vi "COD电极校准.vi"() -> ()   [LabVIEW 2016, in "斯坦道多参数.lvlib"]
uses:
  <vilib>/Utility/miscctls.llb/LVPointTypeDef.ctl
  <vilib>/Utility/miscctls.llb/LVPositionTypeDef.ctl
  <vilib>/Analysis/NI_AALBase.lvlib
panel:
  out "COD水样校正值":dbl format="%#.2f"
  out "浊度测量值":dbl format="%#.2f"
  out "浊度信号值":dbl format="%#.2f"
  out "滤波设定":dbl
  in  "刷新按钮":bool
  out "第三点信号值":dbl
  out "第二点信号值":dbl
  out "第一点信号值":dbl
  out "温度":dbl format="%#.2f"
  out "通讯状态":string
  out "第三点校准值":dbl
  out "标液3":dbl
  out "第二点校准值":dbl
  out "第一点校准值":dbl
  in  "校准停止":bool
  in  "校准启动":bool
  in  "校准模式":u16(ring) items=["两点校准", "单点校准", "三点校准"]
  out "最小值":sgl format="%#.2f"
  out "最大值":sgl format="%#.2f"
  out "波形图表":sgl(graph) caption="历史曲线"
  out "mean":dbl caption="均值" format="%#.2f"
  out "standard deviation":dbl caption="标准差" format="%#.2f"
  out "变异系数":dbl format="%#.6f"
  out "COD测量值":dbl format="%#.2f"
  out "提示":string
  out "标液2":dbl
  out "标液1":dbl
  out "COD信号值":dbl format="%#.2f"
  out "COD偏移修正值":dbl format="%#.2f"
  # "COD电极设定"
  # "℃"
  # "请选择校准模式:"
  # "mg/L"
  # "mg/L"
  # "mg/L"
  # "mg/L"
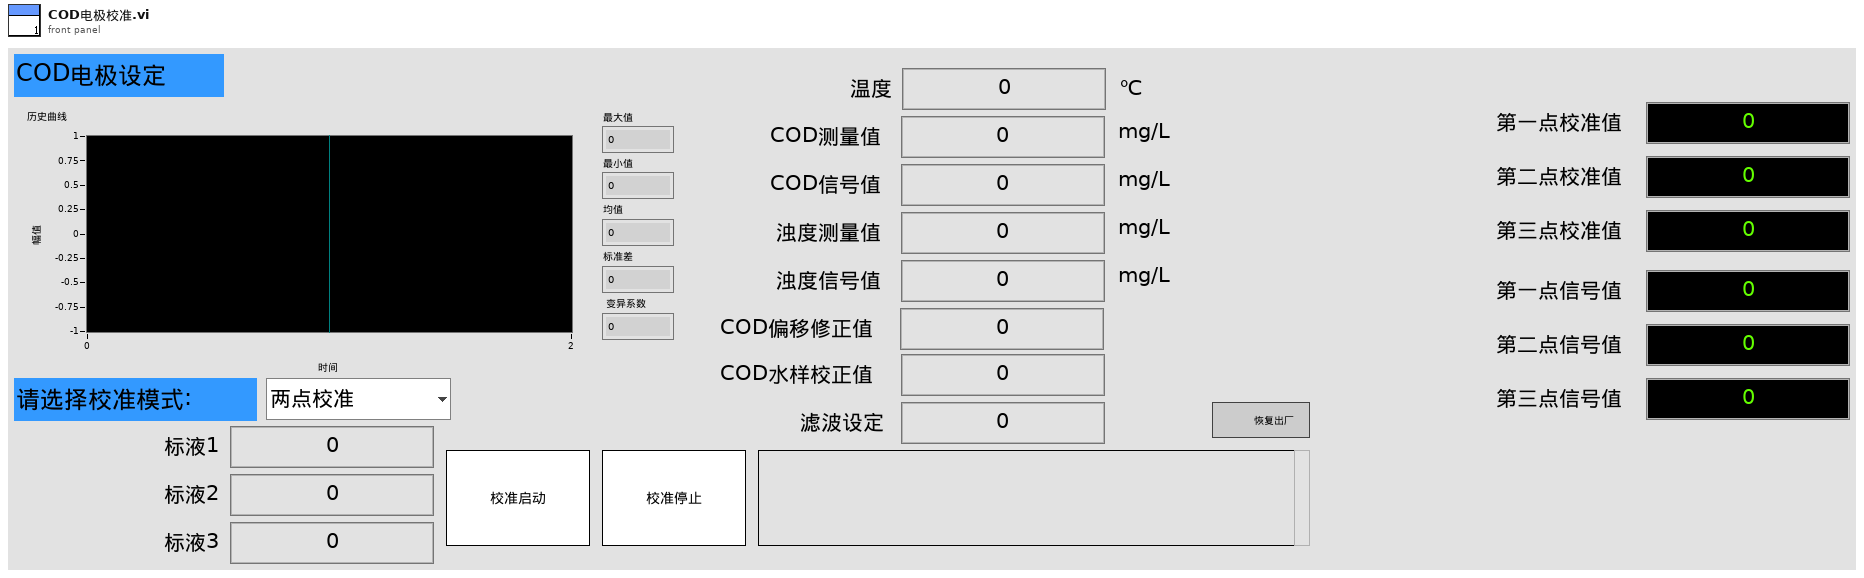
[diagram p1: front panel]
types:
  T1 = enum16{"pH", "DO", "Cond", "Turb", "ORP", "叶绿素a", "藻密度", "COD"}
  T2 = typedef "LVPointTypeDef.ctl" = cluster{"Horizontal":i16, "Vertical":i16}
  T3 = cluster{"电极状态标志":u16, "电极型号标志":u16, "COD测量值":sgl, "浊度测量值":sgl, "COD信号值":sgl, "浊度信号值":sgl, "温度测量值":sgl, "COD偏移修正值":sgl, "浊度偏移修正值":sgl, "COD水样校正值":sgl, "温度偏移修正值":sgl, "COD零点系数":sgl, "COD斜率系数":sgl, "浊度零点系数":sgl, "浊度斜率系数":sgl, "COD测值K值":sgl, "浊度测值K值":sgl, "浊度补偿COD系数值":sgl, "COD温度补偿系数值 ":sgl, "测量周期":u16, "清洗周期":u16, "命令寄存器":u16, "数字滤波设定":u16, "温度模式":enum16{"AUTO", "OFF"}, "生产批次":u16, "电极序号":u16, "串口地址":u16, "串口波特率":enum16{"9600", "19200", "115200"}, "串口校验位":enum16{"NONE", "ODD", "EVEN"}, "串口停止位":enum16{"1bit", "2bit"}, "第一点校正指令":u16, "第一点标准值":sgl, "第二点校正指令":u16, "第二点标准值":sgl, "第三点校正指令":u16, "第三点标准值":sgl, "COD吸光度":sgl, "浊度吸光度":sgl, "温度信号值":sgl}
  T4 = typedef "LVPositionTypeDef.ctl" = cluster{"Left":i32, "Top":i32}
  T5 = enum8{"Enabled", "Disabled", "Disabled and Grayed Out"}
  T6 = cluster{"测量量程":dbl, "测量精度":dbl, "测量间隔":dbl, "消解温度":dbl, "消解时长":dbl, "空白校准时间":timestamp, "曲线截距":dbl, "曲线斜率":dbl, "测量检出限":dbl, "测量信号值":dbl, "线性相关系数":dbl, "二次多项式系数":dbl, "标样校准时间":timestamp, "稀释倍数":dbl, "三项式系数":dbl, "空白标定系数":dbl, "量程系数":dbl, "F0/ORPA":dbl, "F1/ORPB":dbl, "F2/ORPK":dbl, "F3":dbl, "F4":dbl, "F5":dbl, "F6":dbl, "F7":dbl, "X0/滴定数":dbl, "量程":dbl}
  T7 = cluster{"ph":bool, "DO":bool, "Cond":bool, "Turb":bool, "叶绿素a":bool, "藻密度":bool, "ORP":bool, "COD":bool}
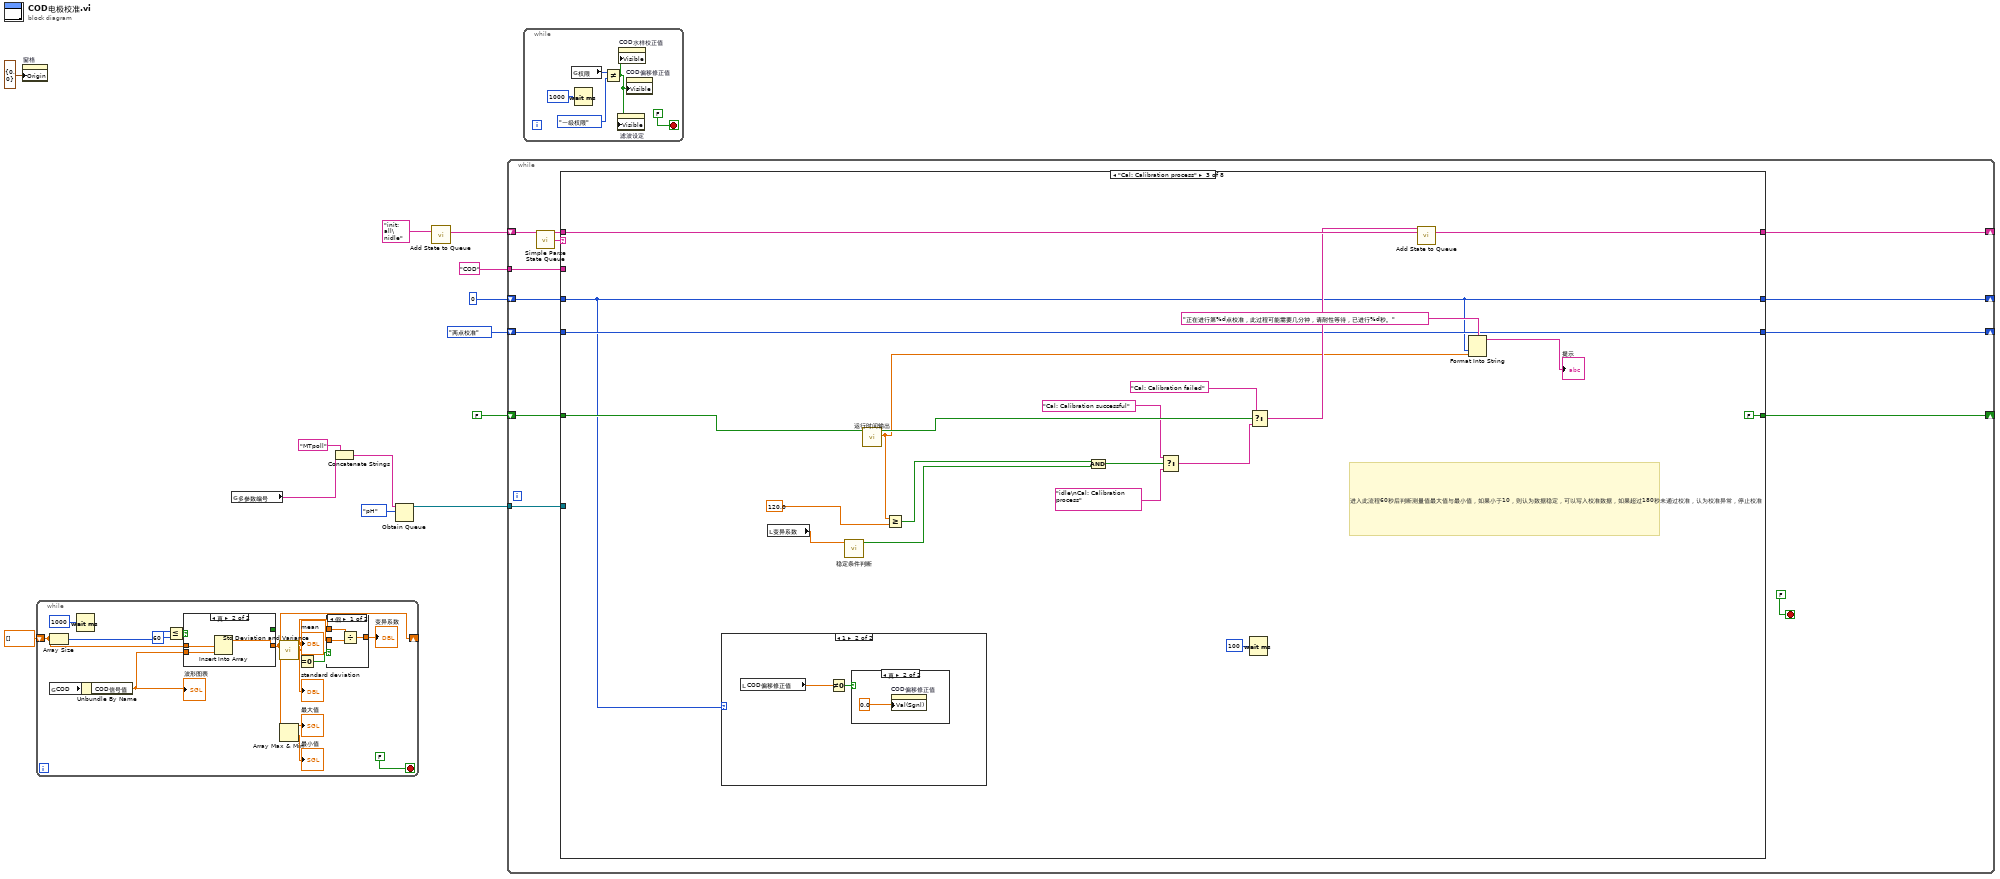
[diagram p0: block diagram]
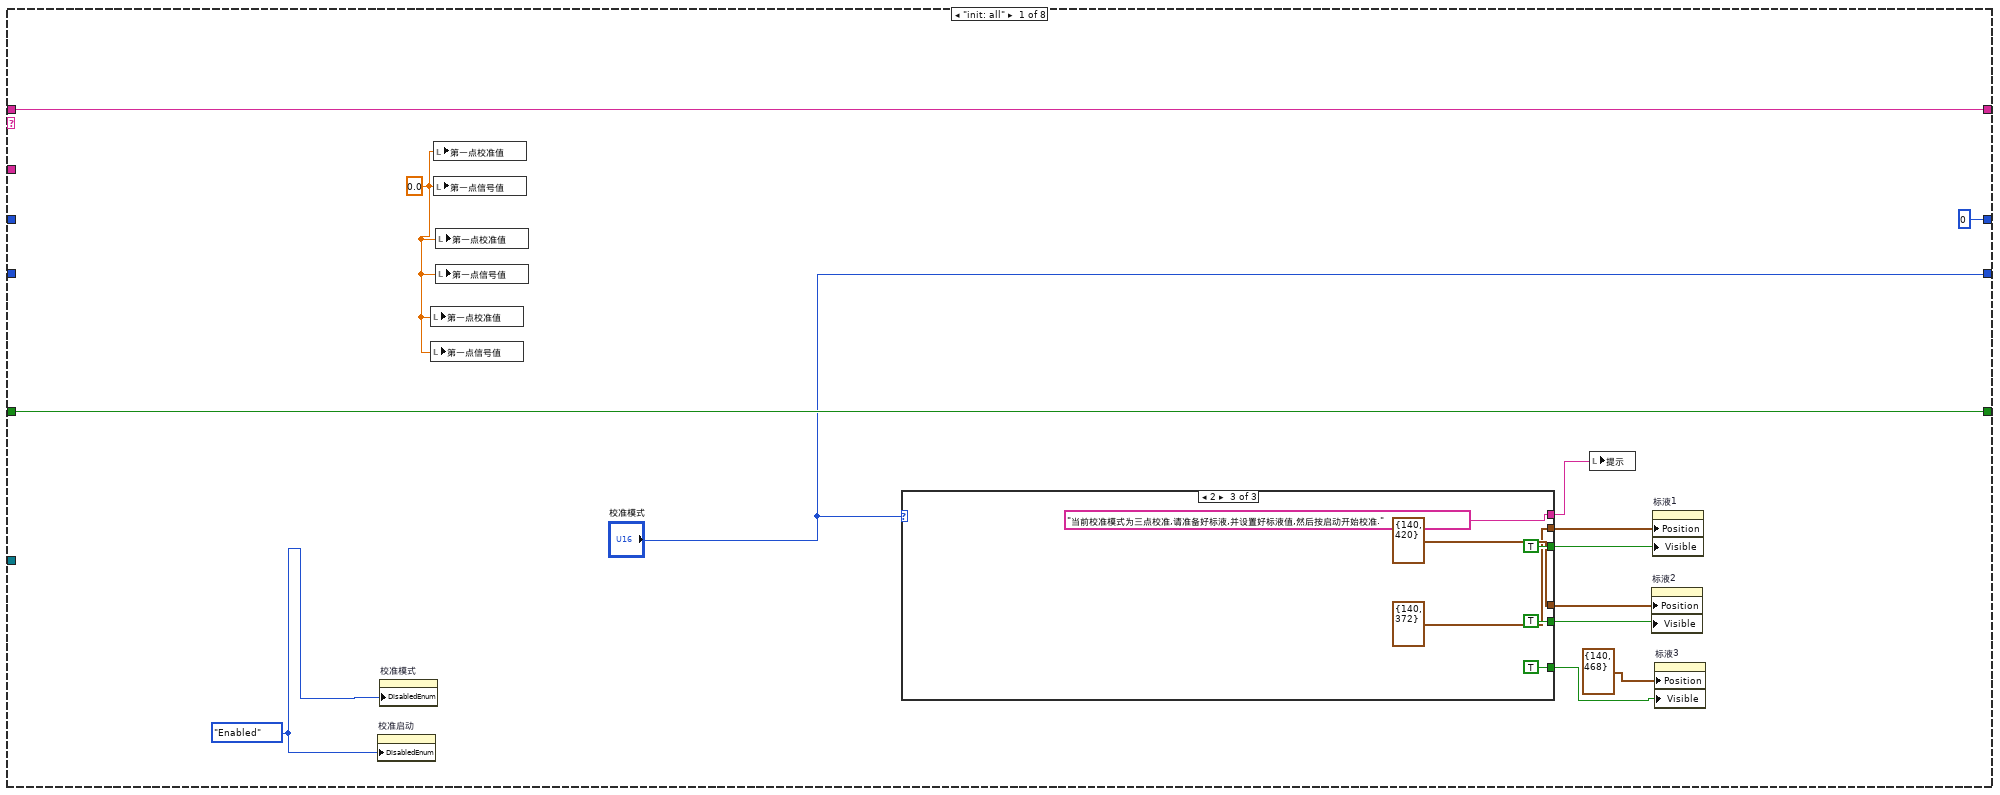
[diagram p2: hidden frame]
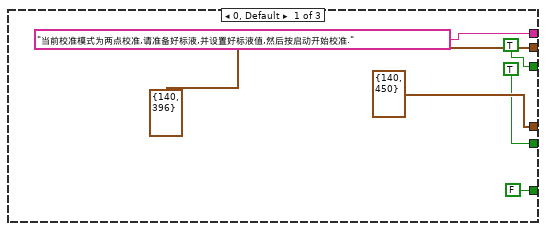
[diagram p3: hidden frame]
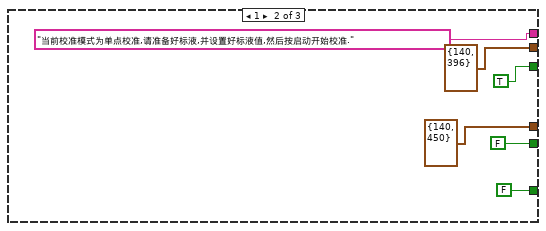
[diagram p4: hidden frame]
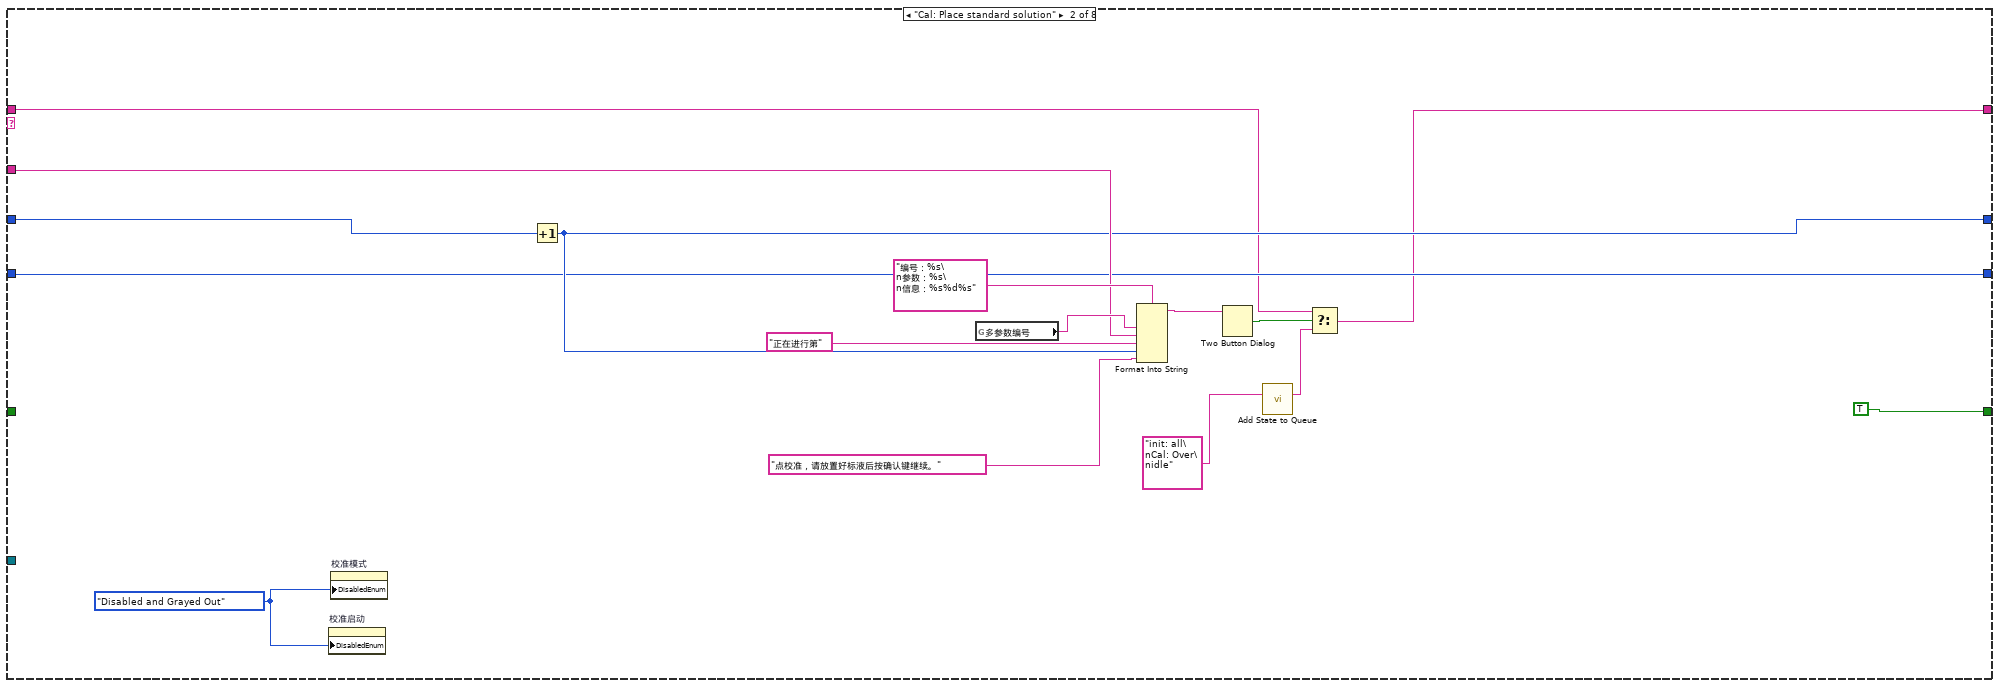
[diagram p5: hidden frame]
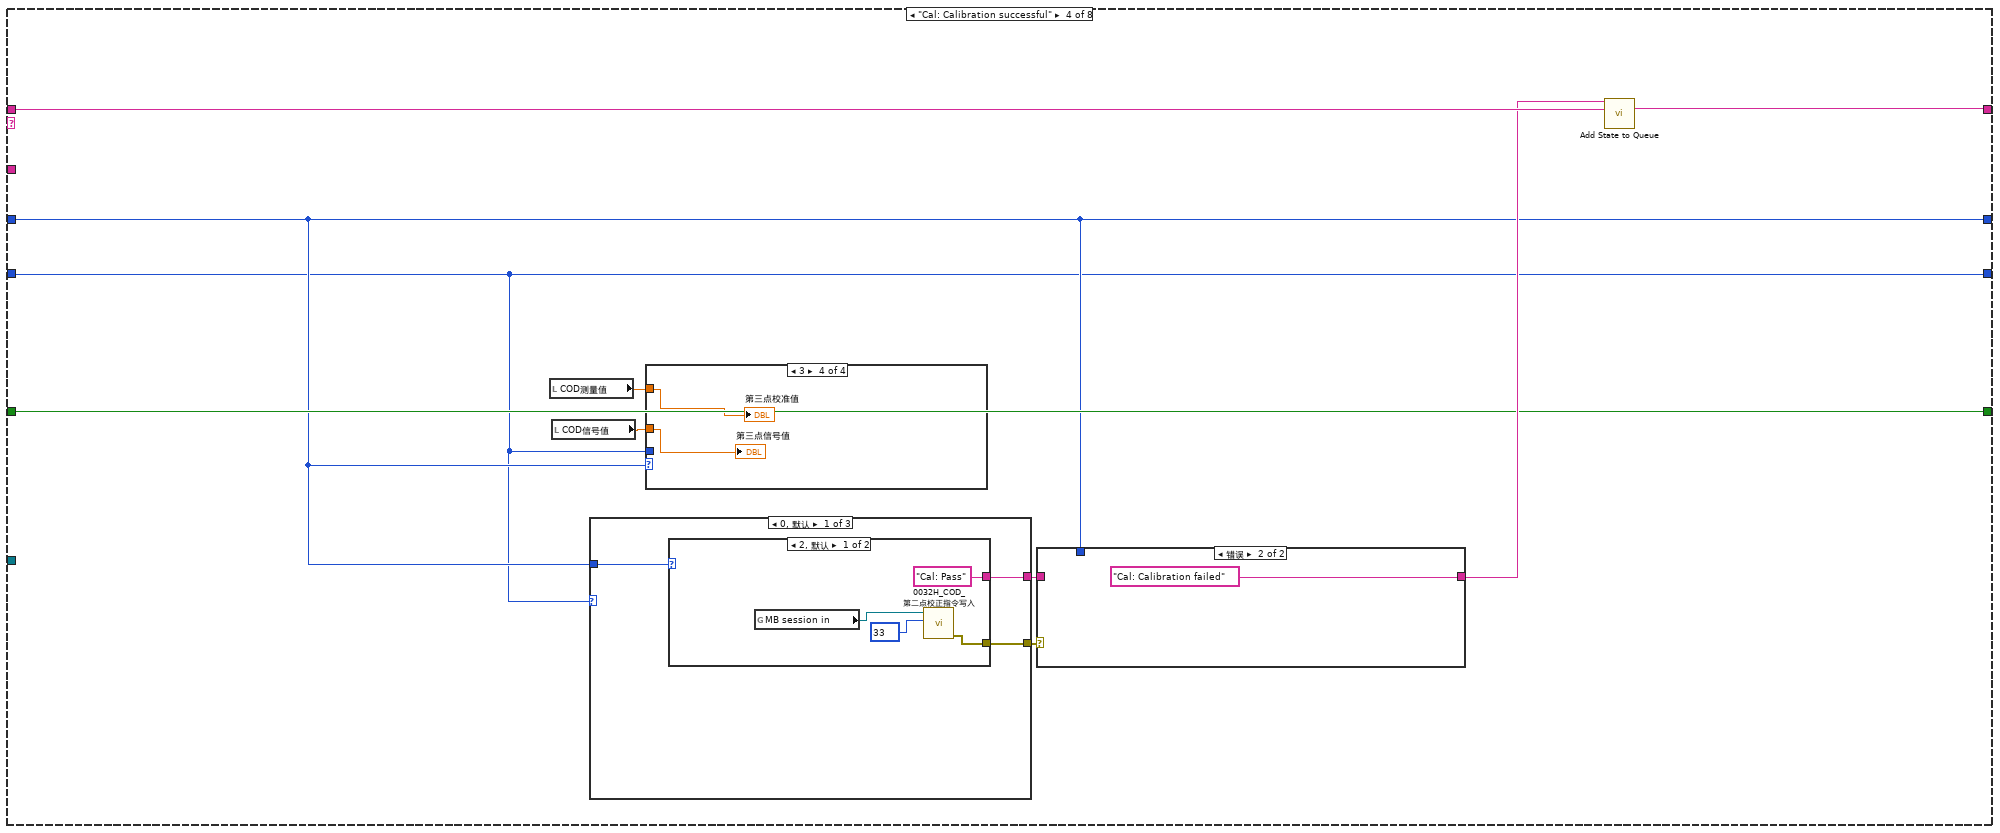
[diagram p8: hidden frame]
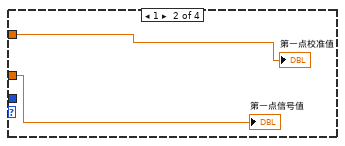
[diagram p10: hidden frame]
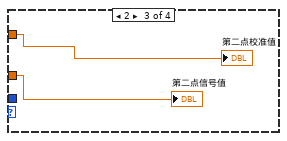
[diagram p11: hidden frame]
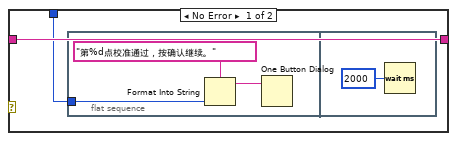
[diagram p12: hidden frame]
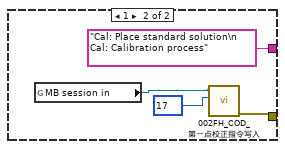
[diagram p13: hidden frame]
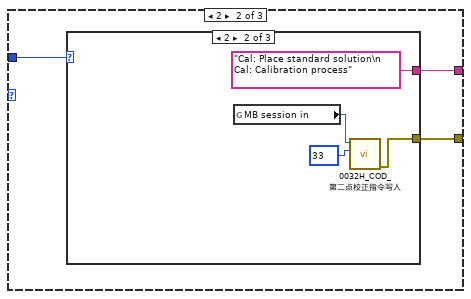
[diagram p14: hidden frame]
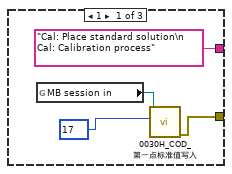
[diagram p15: hidden frame]
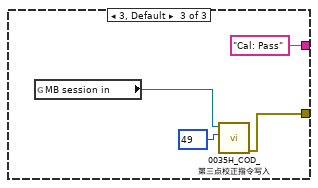
[diagram p16: hidden frame]
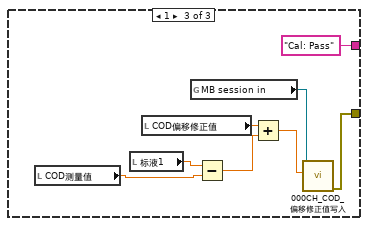
[diagram p17: hidden frame]
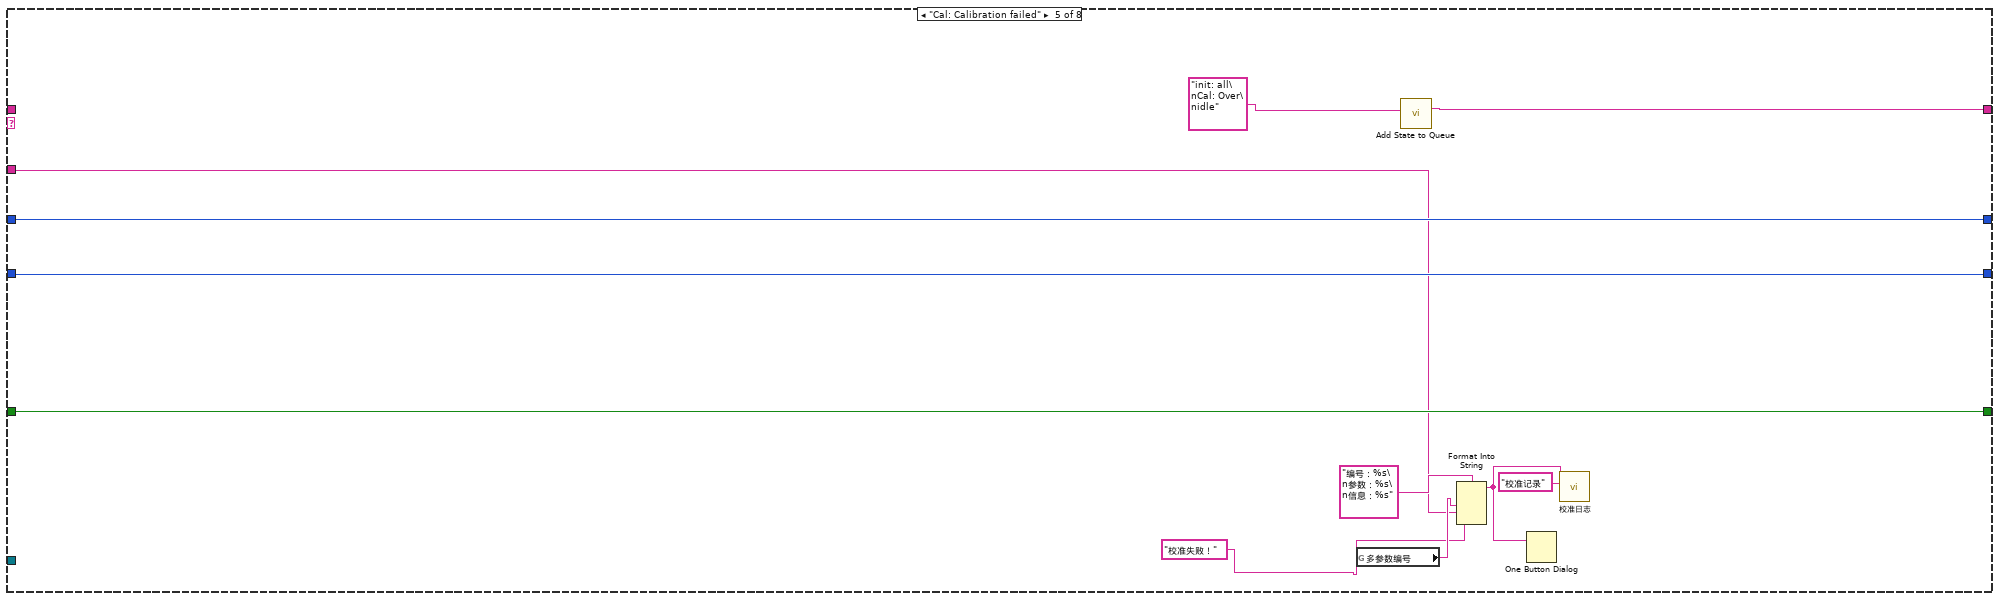
[diagram p18: hidden frame]
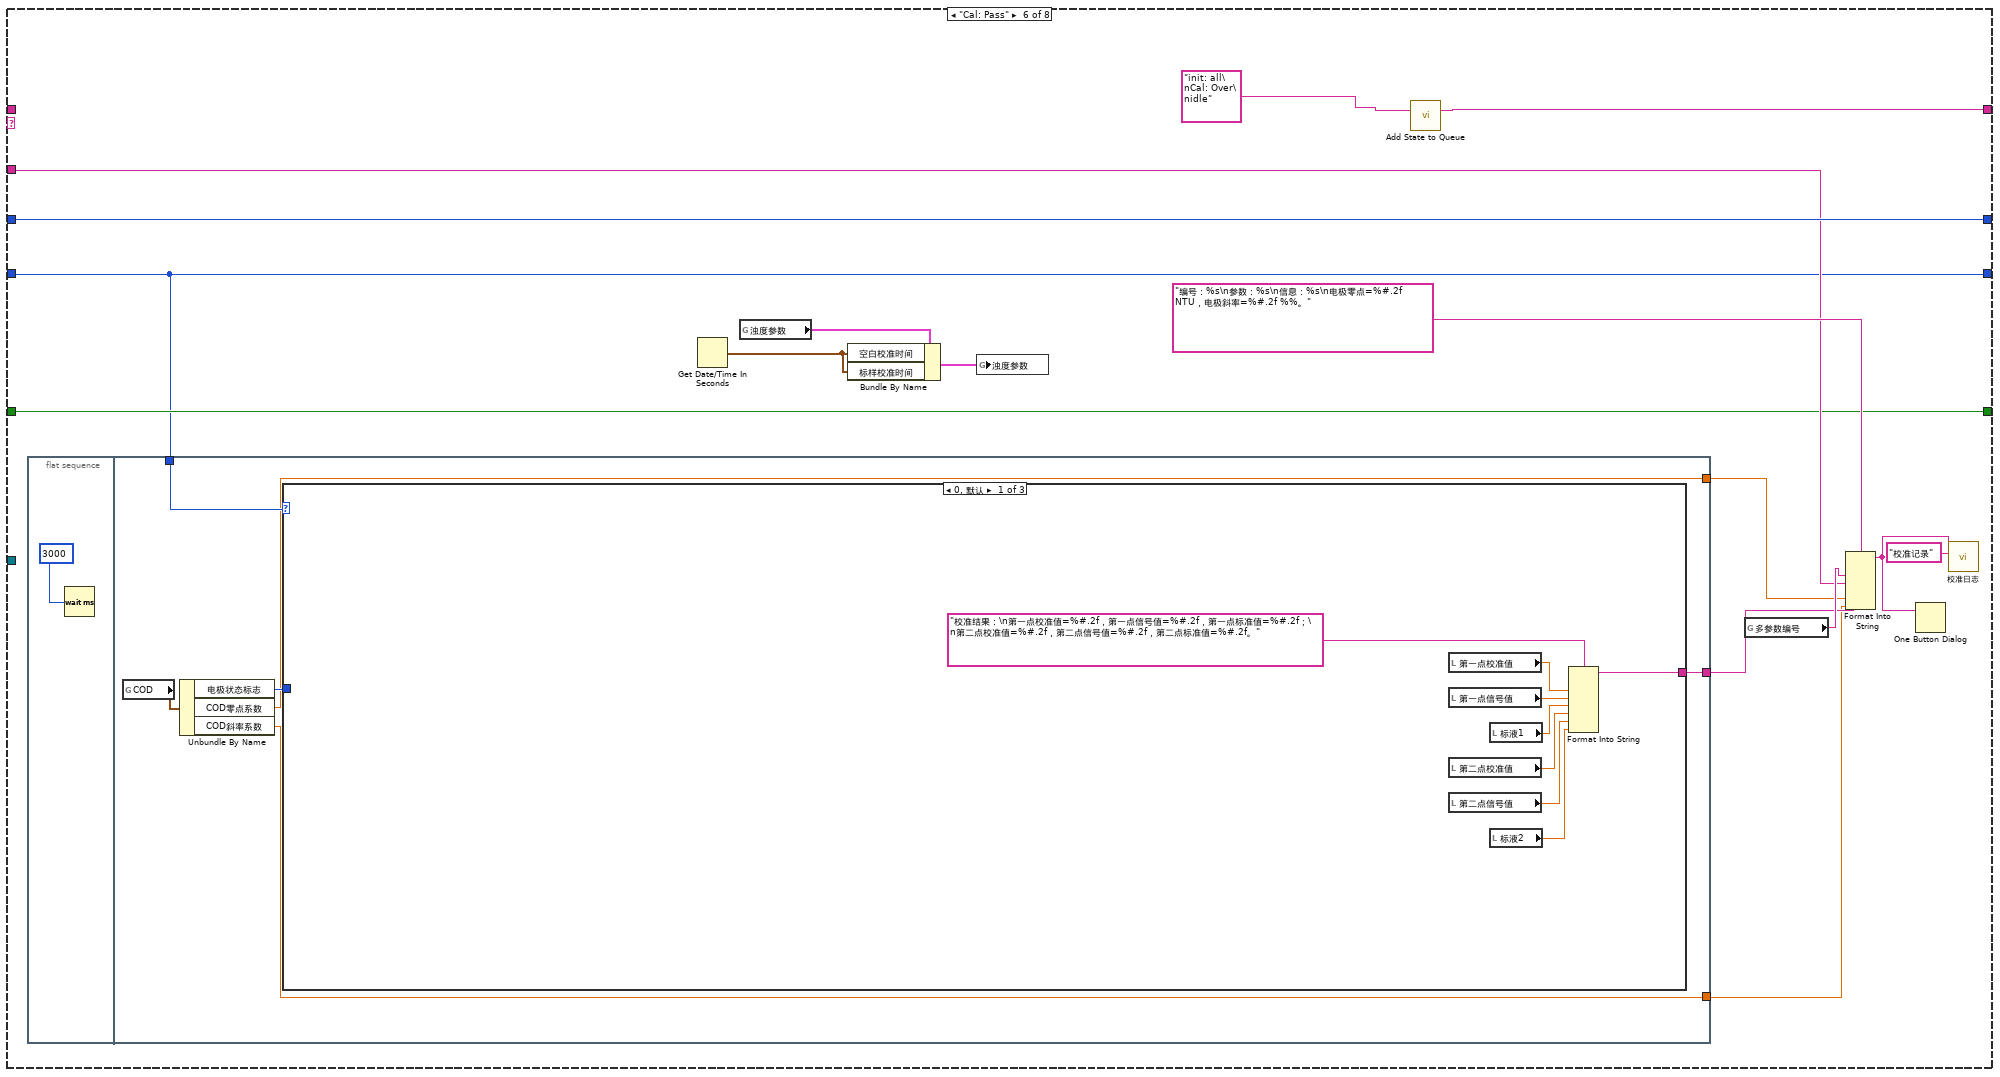
[diagram p19: hidden frame]
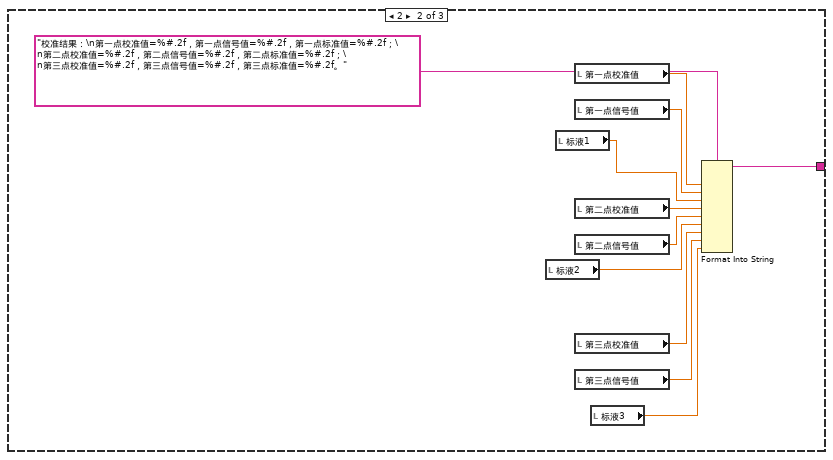
[diagram p20: hidden frame]
diagram:
  n1 = property on="窗格" class="Pane"("Origin"=T2 {"Horizontal"=0, "Vertical"=0} ("原点")) -> ()  [unwired: 2 in, 2 out]
  n2 = while {
    shift-right: [w17] -> _
    shift-left: sgl[] [] -> [w24]
    stop <- FALSE stop-if-true
    n3 = Array Size(array=w24) -> (size(s)=w26:i32)
    n4 = global read "国弘过程全局变量.vi" "COD"() -> (w18:T3)
    n5 = Wait (ms)(milliseconds to wait=u32 1000 ("等待时间（毫秒）")) -> ()  [unwired: 1 out]
    n6 = Unbundle By Name(w18) -> ("COD信号值"=w14:sgl)
    "波形图表" <- w14
    n7 = Less Or Equal?(x=w26, y=60) -> (x <= y?=w25:bool)
    n8 = case shown="真" w25 {
      tunnel: w24 -> [w37 w40]
      tunnel: w14 -> [w35 w39]
      tunnel: [w33 w38] -> w17
      tunnel: [TRUE _] -> _
      frame False {
        n9 = Replace Array Subset(array=w37, new element=w35) -> (w36:sgl[])  [unwired: 1 in]
        n10 = Rotate 1D Array(1:w36, 2:-1 ("n")) -> (0:w33:sgl[])
      }
      frame True {
        n11 = Insert Into Array(array=w40, new element=w39) -> (w38:sgl[])  [unwired: 1 in]
      }
    }
    n12 = call <vilib>:"Std Deviation and Variance.vi"("X"=w17) -> ("mean"=w22:dbl, "standard deviation"=w21:dbl)  [unwired: 1 in, 1 out]
    "mean" <- w22
    "standard deviation" <- w21
    n13 = Array Max & Min(array=w17) -> (max value=→"最大值":sgl, min value=→"最小值":sgl)  [unwired: 2 out]
    n14 = Equal To 0?(x=w22) -> (x = 0?=w23:bool)
    n15 = case shown="假" w23 {
      tunnel: w21 -> [w31 _]
      tunnel: [w30 _] -> w20
      tunnel: w22 -> [w29 _]
      frame False {
        n16 = Divide(x=w31, y=w29) -> (x/y=w30:dbl)
      }
      frame True {
      }
    }
    "变异系数" <- w20
  }
  n17 = global read "多参数全局变量.vi" "多参数编号"() -> (w2:string)
  n18 = Concatenate Strings("MTpoll" ("名称（未命名）"), w2) -> (w4:string)
  n19 = Obtain Queue(name (unnamed)=w4, element data type=T1."pH" ("枚举")) -> (queue out=w1:refnum<queue>)  [unwired: 3 in, 2 out]
  n20 = call "Add State to Queue.vi"("State(s) In (\"\")"="init: all\nidle" ("State(s) In (\"\")")) -> ("States Out"=w10:string)  [unwired: 14 in]
  n21 = while {
    shift-right: [w49] -> _
    shift-left: w10 -> [w53]
    shift-right: [w46] -> _
    shift-left: 0 -> [w48]
    tunnel: "COD" ("State(s) In (\"\")") -> [w47]
    shift-right: [w44] -> _
    shift-left: enum16{"两点校准", "单点校准", "三点校准"}."两点校准" ("校准模式") -> [w45]
    shift-right: [w42] -> _
    shift-left: FALSE -> [w43]
    tunnel: w1 -> [w41]
    stop <- FALSE stop-if-true
    n22 = call "Simple Parse State Queue.vi"("State Queue"=w53) -> ("Remain States"=w50:string, "Next State"=w51:string)  [unwired: 13 in]
    n23 = case shown="\"Cal: Calibration process\"" w51 {
      tunnel: w50 -> [w66 w88 w120 w132 _ _ w243 w254]
      tunnel: [w66 w87 w119 w131 w189 w199 w243 w253] -> w49
      tunnel: w48 -> [_ w96 w105 w126 w192 w208 w242 w251]
      tunnel: w47 -> [_ w97 _ _ w183 w204 _ _]
      tunnel: [0 w94 w105 w126 w192 w208 w242 w252] -> w46
      tunnel: w45 -> [_ w93 w106 w125 w191 w200 w241 w250]
      tunnel: ["校准模式" w93 w106 w125 w191 w200 w241 w250] -> w44
      tunnel: w43 -> [w63 _ w108 w127 w190 w203 w240 w248]
      tunnel: [w63 TRUE FALSE w127 w190 w203 w240 w248] -> w42
      tunnel: w41 -> [_ _ _ _ _ _ _ w247]
      frame "init: all" {
        w61 = T5."Enabled" ("禁用")
        w62 = 0.0 ("第一点校准值")
        n24 = property on="校准启动" class="Bool"("DisabledEnum"=w61) -> ()  [unwired: 2 in, 2 out]
        n25 = property on="校准模式" class="Ring (严格)"("DisabledEnum"=w61) -> ()  [unwired: 2 in, 2 out]
        n26 = local write "第一点校准值"(w62) -> ()
        n27 = local write "第一点信号值"(w62) -> ()
        n28 = local write "第一点校准值"(w62) -> ()
        n29 = local write "第一点信号值"(w62) -> ()
        n30 = local write "第一点校准值"(w62) -> ()
        n31 = local write "第一点信号值"(w62) -> ()
        n32 = case shown="2" "校准模式" {
          tunnel: ["当前校准模式为两点校准,请准备好标液,并设置好标液值,然后按启动开始校准." ("提示") "当前校准模式为单点校准,请准备好标液,并设置好标液值,然后按启动开始校准." ("提示") "当前校准模式为三点校准,请准备好标液,并设置好标液值,然后按启动开始校准." ("提示")] -> w65
          tunnel: [T4 {"Left"=140, "Top"=396} ("位置") T4 {"Left"=140, "Top"=396} ("位置") T4 {"Left"=140, "Top"=372} ("位置")] -> w59
          tunnel: [TRUE ("可见") TRUE ("可见") TRUE ("可见")] -> w58
          tunnel: [FALSE ("可见") FALSE ("可见") TRUE ("可见")] -> w56
          tunnel: [TRUE ("可见") FALSE ("可见") TRUE ("可见")] -> w55
          tunnel: [T4 {"Left"=140, "Top"=450} ("位置 2") T4 {"Left"=140, "Top"=450} ("位置 2") T4 {"Left"=140, "Top"=420} ("位置 2")] -> w54
          frame 0, Default {
          }
          frame 1 {
          }
          frame 2 {
          }
        }
        n33 = local write "提示"(w65) -> ()
        n34 = property on="标液2" class="DigNum (严格)"("Position"=w54, "Visible"=w55) -> ()  [unwired: 2 in, 2 out]
        n35 = property on="标液1" class="DigNum (严格)"("Position"=w59, "Visible"=w58) -> ()  [unwired: 2 in, 2 out]
        n36 = property on="标液3" class="DigNum (严格)"("Position"=T4 {"Left"=140, "Top"=468} ("位置 3"), "Visible"=w56) -> ()  [unwired: 2 in, 2 out]
      }
      frame "Cal: Place standard solution" {
        w86 = T5."Disabled and Grayed Out" ("禁用")
        n37 = property on="校准启动" class="Bool"("DisabledEnum"=w86) -> ()  [unwired: 2 in, 2 out]
        n38 = property on="校准模式" class="Ring (严格)"("DisabledEnum"=w86) -> ()  [unwired: 2 in, 2 out]
        n39 = Increment(x=w96) -> (x+1=w94:i32)
        n40 = global read "多参数全局变量.vi" "多参数编号"() -> (w99:string)
        n41 = Format Into String(format string="编号：%s\n参数：%s\n信息：%s%d%s" ("格式字符串"), w99, w97, "正在进行第" ("消息"), w94, "点校准，请放置好标液后按确认键继续。" ("消息")) -> (resulting string=w91:string)  [unwired: 2 in, 1 out]
        n42 = Two Button Dialog(message=w91) -> (T button?=w90:bool)  [unwired: 2 in]
        n43 = call "Add State to Queue.vi"("State(s) In (\"\")"="init: all\nCal: Over\nidle" ("State(s) In (\"\")")) -> ("States Out"=w89:string)  [unwired: 14 in]
        n44 = Select(t=w88, s=w90, f=w89) -> (s? t:f=w87:string)
      }
      frame "Cal: Calibration process" {
        # "进入此流程60秒后判断测量值最大值与最小值，如果小于10，则认为数据稳定，可以写入校准数据，如果超过180秒未通过校准，认为校准异常，停止校准"
        n45 = case shown="1" w105 {
          frame 0, Default {
          }
          frame 1 {
            n46 = local read "COD偏移修正值"() -> (w122:dbl)
            n47 = Not Equal To 0?(x=w122) -> (x != 0?=w123:bool)
            n48 = case shown="真" w123 {
              frame False {
              }
              frame True {
                n49 = property on="COD偏移修正值" class="DigNum (严格)"("Val(Sgnl)"=0.0 ("值(信号)")) -> ()  [unwired: 2 in, 2 out]
              }
            }
          }
        }
        n50 = local read "变异系数"() -> (w102:dbl)
        n51 = call "稳定条件判断.vi"("变异系数"=w102) -> ("布尔"=w101:bool)  [unwired: 10 in]
        n52 = call "运行时间输出.vi"("初始化"=w108) -> ("Elapsed Time (s)"=w104:dbl, "Time has Elapsed"=w121:bool)  [unwired: 9 in]
        n53 = Greater Or Equal?(x=w104, y=120.0) -> (x >= y?=w116:bool)
        n54 = And(x=w116, y=w101) -> (x .and. y?=w113:bool)
        n55 = Select(t="Cal: Calibration successful" ("State(s) In (\"\")"), s=w113, f="idle\nCal: Calibration process" ("State(s) In (\"\")")) -> (s? t:f=w112:string)
        n56 = Wait (ms)(milliseconds to wait=u32 100 ("等待时间（毫秒）")) -> ()  [unwired: 1 out]
        n57 = Select(t="Cal: Calibration failed" ("State(s) In (\"\")"), s=w121, f=w112) -> (s? t:f=w111:string)
        n58 = call "Add State to Queue.vi"("State(s) In Front (\"\")"=w111, "State(s) In (\"\")"=w120) -> ("States Out"=w119:string)  [unwired: 13 in]
        n59 = Format Into String(format string="正在进行第%d点校准，此过程可能需要几分钟，请耐性等待，已进行%d秒。" ("格式字符串"), w105, w104) -> (resulting string=→"提示":string)  [unwired: 2 in, 1 out]
      }
      frame "Cal: Calibration successful" {
        n60 = local read "COD测量值"() -> (w128:dbl)
        n61 = local read "COD信号值"() -> (w129:dbl)
        n62 = case shown="0, 默认" w125 {
          tunnel: [w150 w161 w174] -> w134
          tunnel: [w149 w159 "Cal: Pass" ("State(s) In (\"\")")] -> w133
          tunnel: w126 -> [w148 w160 _]
          frame 0, Default {
            n63 = case shown="2, 默认" w148 {
              tunnel: [w153 w157] -> w150
              tunnel: ["Cal: Pass" ("State(s) In (\"\")") "Cal: Place standard solution\n Cal: Calibration process" ("State(s) In (\"\")")] -> w149
              frame 2, Default {
                n64 = global read "多参数全局变量.vi" "MB session in"() -> (w152:refnum<class "MB_Master.lvclass">)
                n65 = call "0032H_COD_第二点校正指令写入.vi"("数值"=u16 33, "MB session in"=w152) -> ("error out"=w153:errorcluster)  [unwired: 8 in, 1 out]
              }
              frame 1 {
                n66 = global read "多参数全局变量.vi" "MB session in"() -> (w156:refnum<class "MB_Master.lvclass">)
                n67 = call "002FH_COD_第一点校正指令写入.vi"("数值"=u16 17, "MB session in"=w156) -> ("error out"=w157:errorcluster)  [unwired: 8 in, 1 out]
              }
            }
          }
          frame 2 {
            n68 = case shown="2" w160 {
              tunnel: [w164 w167 w171] -> w161
              tunnel: ["Cal: Place standard solution\n Cal: Calibration process" ("State(s) In (\"\")") "Cal: Place standard solution\n Cal: Calibration process" ("State(s) In (\"\")") "Cal: Pass" ("State(s) In (\"\")")] -> w159
              frame 1 {
                n69 = global read "多参数全局变量.vi" "MB session in"() -> (w163:refnum<class "MB_Master.lvclass">)
                n70 = call "0030H_COD_第一点标准值写入.vi"("数值"=u16 17, "MB session in"=w163) -> ("error out"=w164:errorcluster)  [unwired: 8 in, 1 out]
              }
              frame 2 {
                n71 = global read "多参数全局变量.vi" "MB session in"() -> (w166:refnum<class "MB_Master.lvclass">)
                n72 = call "0032H_COD_第二点校正指令写入.vi"("数值"=u16 33, "MB session in"=w166) -> ("error out"=w167:errorcluster)  [unwired: 8 in, 1 out]
              }
              frame 3, Default {
                n73 = global read "多参数全局变量.vi" "MB session in"() -> (w170:refnum<class "MB_Master.lvclass">)
                n74 = call "0035H_COD_第三点校正指令写入.vi"("数值"=u16 49, "MB session in"=w170) -> ("error out"=w171:errorcluster)  [unwired: 8 in, 1 out]
              }
            }
          }
          frame 1 {
            n75 = local read "COD测量值"() -> (w177:dbl)
            n76 = local read "标液1"() -> (w181:dbl)
            n77 = local read "COD偏移修正值"() -> (w179:dbl)
            n78 = global read "多参数全局变量.vi" "MB session in"() -> (w176:refnum<class "MB_Master.lvclass">)
            n79 = Subtract(x=w181, y=w177) -> (x-y=w180:dbl)
            n80 = Add(x=w179, y=w180) -> (x+y=w175:dbl)
            n81 = call "000CH_COD_偏移修正值写入.vi"("数值"=w175, "MB session in"=w176) -> ("error out"=w174:errorcluster)  [unwired: 8 in, 1 out]
          }
        }
        n82 = case shown="3" w126 {
          tunnel: w129 -> [_ w136 w138 w140]
          tunnel: w128 -> [_ w135 w137 w139]
          tunnel: w125 -> [_ _ _ _]
          frame 0, Default {
          }
          frame 1 {
            "第一点信号值" <- w136
            "第一点校准值" <- w135
          }
          frame 2 {
            "第二点信号值" <- w138
            "第二点校准值" <- w137
          }
          frame 3 {
            "第三点信号值" <- w140
            "第三点校准值" <- w139
          }
        }
        n83 = case shown="错误" w134 {
          tunnel: w133 -> [w142 _]
          tunnel: [w142 "Cal: Calibration failed" ("State(s) In (\"\")")] -> w130
          tunnel: w126 -> [w141 _]
          frame No Error {
            n84 = flat-sequence {
              tunnel: w141 -> [w143]
              frame #0 {
                n85 = Format Into String(format string="第%d点校准通过，按确认继续。" ("格式字符串"), w143) -> (resulting string=w145:string)  [unwired: 2 in, 1 out]
                n86 = One Button Dialog(message=w145) -> ()  [unwired: 1 in, 1 out]
              }
              frame #1 {
                n87 = Wait (ms)(milliseconds to wait=u32 2000 ("等待时间（毫秒）")) -> ()  [unwired: 1 out]
              }
            }
          }
          frame Error {
          }
        }
        n88 = call "Add State to Queue.vi"("State(s) In Front (\"\")"=w130, "State(s) In (\"\")"=w132) -> ("States Out"=w131:string)  [unwired: 13 in]
      }
      frame "Cal: Calibration failed" {
        n89 = global read "多参数全局变量.vi" "多参数编号"() -> (w186:string)
        n90 = call "Add State to Queue.vi"("State(s) In (\"\")"="init: all\nCal: Over\nidle" ("State(s) In (\"\")")) -> ("States Out"=w189:string)  [unwired: 14 in]
        n91 = Format Into String(format string="编号：%s\n参数：%s\n信息：%s" ("格式字符串"), w186, w183, "校准失败！" ("消息")) -> (resulting string=w185:string)  [unwired: 2 in, 1 out]
        n92 = One Button Dialog(message=w185) -> ()  [unwired: 1 in, 1 out]
        n93 = call "校准日志.vi"("table"="校准记录", "日志信息"=w185) -> ()  [unwired: 9 in, 1 out]
      }
      frame "Cal: Pass" {
        n94 = flat-sequence {
          tunnel: [w213] -> w201
          tunnel: w200 -> [w212]
          tunnel: [w211] -> w198
          tunnel: [w210] -> w197
          frame #0 {
            n95 = Wait (ms)(milliseconds to wait=u32 3000 ("等待时间（毫秒）")) -> ()  [unwired: 1 out]
          }
          frame #1 {
            n96 = global read "国弘过程全局变量.vi" "COD"() -> (w214:T3)
            n97 = Unbundle By Name(w214) -> ("电极状态标志"=w215:u16, "COD零点系数"=w211:sgl, "COD斜率系数"=w210:sgl)
            n98 = case shown="0, 默认" w212 {
              tunnel: [w223 w234 w239] -> w213
              tunnel: w215 -> [_ _ _]
              frame 0, Default {
                n99 = local read "第一点校准值"() -> (w221:dbl)
                n100 = local read "第一点信号值"() -> (w222:dbl)
                n101 = local read "第二点校准值"() -> (w218:dbl)
                n102 = local read "第二点信号值"() -> (w217:dbl)
                n103 = local read "标液1"() -> (w219:dbl)
                n104 = local read "标液2"() -> (w216:dbl)
                n105 = Format Into String(format string="校准结果：\n第一点校准值=%#.2f，第一点信号值=%#.2f，第一点标准值=%#.2f；\n第二点校准值=%#.2f，第二点信号值=%#.2f，第二点标准值=%#.2f。" ("提示"), w221, w222, w219, w218, w217, w216) -> (resulting string=w223:string)  [unwired: 2 in, 1 out]
              }
              frame 2 {
                n106 = local read "标液2"() -> (w225:dbl)
                n107 = local read "标液1"() -> (w226:dbl)
                n108 = local read "第一点校准值"() -> (w233:dbl)
                n109 = local read "第一点信号值"() -> (w231:dbl)
                n110 = local read "第二点校准值"() -> (w230:dbl)
                n111 = local read "第二点信号值"() -> (w229:dbl)
                n112 = local read "第三点校准值"() -> (w228:dbl)
                n113 = local read "第三点信号值"() -> (w227:dbl)
                n114 = local read "标液3"() -> (w224:dbl)
                n115 = Format Into String(format string="校准结果：\n第一点校准值=%#.2f，第一点信号值=%#.2f，第一点标准值=%#.2f；\n第二点校准值=%#.2f，第二点信号值=%#.2f，第二点标准值=%#.2f；\n第三点校准值=%#.2f，第三点信号值=%#.2f，第三点标准值=%#.2f。" ("提示"), w233, w231, w226, w230, w229, w225, w228, w227, w224) -> (resulting string=w234:string)  [unwired: 2 in, 1 out]
              }
              frame 1 {
                n116 = local read "第一点校准值"() -> (w238:dbl)
                n117 = local read "第一点信号值"() -> (w236:dbl)
                n118 = local read "标液1"() -> (w235:dbl)
                n119 = Format Into String(format string="校准结果：\n校准值=%#.2f，信号值=%#.2f，标准值=%#.2f。" ("提示"), w238, w236, w235) -> (resulting string=w239:string)  [unwired: 2 in, 1 out]
              }
            }
          }
        }
        n120 = Get Date/Time In Seconds() -> (seconds since 1Jan1904=w193:timestamp)
        n121 = global read "断电保存变量.vi" "浊度参数"() -> (w195:T6)
        n122 = Bundle By Name(cluster=w195, "空白校准时间"=w193, "标样校准时间"=w193) -> (w194:T6)
        n123 = global write "断电保存变量.vi" "浊度参数"(w194) -> ()
        n124 = call "Add State to Queue.vi"("State(s) In (\"\")"="init: all\nCal: Over\nidle" ("State(s) In (\"\")")) -> ("States Out"=w199:string)  [unwired: 14 in]
        n125 = global read "多参数全局变量.vi" "多参数编号"() -> (w205:string)
        n126 = Format Into String(format string="编号：%s\n参数：%s\n信息：%s\n电极零点=%#.2f NTU，电极斜率=%#.2f %%。" ("格式字符串"), w205, w204, w201, w198, w197) -> (resulting string=w202:string)  [unwired: 2 in, 1 out]
        n127 = One Button Dialog(message=w202) -> ()  [unwired: 1 in, 1 out]
        n128 = call "校准日志.vi"("table"="校准记录", "日志信息"=w202) -> ()  [unwired: 9 in, 1 out]
      }
      frame "Cal: Over" {
        n129 = global read "多参数全局变量.vi" "校准运行状态"() -> (w245:T7)
        n130 = Bundle By Name(cluster=w245, "COD"=FALSE ("Turb")) -> (w246:T7)
        n131 = global write "多参数全局变量.vi" "校准运行状态"(w246) -> ()
      }
      frame "idle", Default {
        n132 = event shown="[0] 超时" {
          selector: _ -> [_ _ _ _ _ _ _ _ _ _ _ _]
          dyn-events: _ -> [_ _ _ _ _ _ _ _ _ _ _ _]
          timeout: 10 -> [_ _ _ _ _ _ _ _ _ _ _ _]
          tunnel: [_ _ _ w287 w296 w305 w314 w323 w332 _ _ _] -> _
          tunnel: w254 -> [w273 w277 w282 w293 w302 w306 w315 w324 w336 w343 w352 _]
          tunnel: [w272 w276 w283 w292 w301 w310 w319 w328 w337 w342 w351 w354] -> w253
          tunnel: [w271 w274 w284 w291 w300 w311 w320 w329 w338 w341 w349 w355] -> w252
          tunnel: w251 -> [w271 w274 w284 w291 w300 w311 w320 w329 w338 w341 w349 w355]
          tunnel: w247 -> [_ _ _ w286 w295 w304 w313 w322 w331 _ _ _]
          event Timeout {
            n133 = event-data() -> ()  [unwired: 1 in, 3 out]
            n134 = global read "国弘过程全局变量.vi" "COD"() -> (w260:T3)
            n135 = Unbundle By Name(w260) -> ("数字滤波设定"=→"滤波设定":u16, "COD偏移修正值"=→"COD偏移修正值":sgl, "COD信号值"=→"COD信号值":sgl, "浊度信号值"=→"浊度信号值":sgl, "浊度测量值"=→"浊度测量值":sgl, "第一点标准值"=→"标液1":sgl, "COD水样校正值"=→"COD水样校正值":sgl, "第二点标准值"=→"标液2":sgl, "COD测量值"=→"COD测量值":sgl, "第三点标准值"=→"标液3":sgl, "温度测量值"=→"温度":sgl)  [unwired: 1 out]
            n136 = global read "多参数全局变量.vi" "cod通讯状态"() -> (w269:bool)
            n137 = property on="通讯状态" class="Str"("Blinking"=TRUE ("闪烁"), "Text.BG Color"=u32 16711680, "Visible"=w269) -> ()  [unwired: 2 in, 2 out]
            n138 = call "Add State to Queue.vi"("State(s) In (\"\")"=w273) -> ("States Out"=w272:string)  [unwired: 14 in]
            "通讯状态" <- "通讯异常" ("当前串口")
          }
          event "校准模式": Value Change {
            n139 = event-data() -> ()  [unwired: 1 in, 6 out]
            n140 = call "Add State to Queue.vi"("State(s) In (\"\")"=w277, "State(s) At Back (\"\")"="init: all\nidle" ("State(s) In (\"\")")) -> ("States Out"=w276:string)  [unwired: 13 in]
          }
          event "COD偏移修正值", "标液1", "标液2", "标液3", "滤波设定", "COD水样校正值": Mouse Down {
            n141 = event-data() -> ("CtlRef"=w281:refnum<vi>)  [unwired: 1 in, 7 out]
            n142 = property class="DigNum (严格)"(reference=w281) -> (reference out=w278:refnum<vi>, "Value"=w279:dbl)  [unwired: 1 in, 1 out]
            n143 = call "数字键盘.vi"("OldNumber"=w279) -> ("NewNumber"=w280:dbl)  [unwired: 1 in]
            n144 = property class="DigNum (严格)"(reference=w278, "Val(Sgnl)"=w280) -> ()  [unwired: 1 in, 2 out]
            n145 = call "Add State to Queue.vi"("State(s) In (\"\")"=w282) -> ("States Out"=w283:string)  [unwired: 14 in]
          }
          event "COD偏移修正值": Value Change {
            n146 = event-data() -> ("NewVal"=w288:dbl)  [unwired: 1 in, 5 out]
            n147 = global read "多参数全局变量.vi" "MB session in"() -> (w289:refnum<class "MB_Master.lvclass">)
            n148 = call "000CH_浊度_浊度偏移修正值写入.vi"("数值"=w288, "MB session in"=w289) -> ("error out"=w290:errorcluster)  [unwired: 8 in, 1 out]
            n149 = Enqueue Element At Opposite End(queue=w286, element=T1."COD" ("枚举"), error in (no error)=w290) -> (error out=w287:errorcluster)  [unwired: 1 in, 2 out]
            n150 = call "Add State to Queue.vi"("State(s) In (\"\")"=w293) -> ("States Out"=w292:string)  [unwired: 14 in]
          }
          event "COD水样校正值": Value Change {
            n151 = event-data() -> ("NewVal"=w297:dbl)  [unwired: 1 in, 5 out]
            n152 = global read "多参数全局变量.vi" "MB session in"() -> (w298:refnum<class "MB_Master.lvclass">)
            n153 = call "0010H_COD_水样校正值写入.vi"("数值"=w297, "MB session in"=w298) -> ("error out"=w299:errorcluster)  [unwired: 8 in, 1 out]
            n154 = Enqueue Element At Opposite End(queue=w295, element=T1."COD" ("枚举"), error in (no error)=w299) -> (error out=w296:errorcluster)  [unwired: 1 in, 2 out]
            n155 = call "Add State to Queue.vi"("State(s) In (\"\")"=w302) -> ("States Out"=w301:string)  [unwired: 14 in]
          }
          event "标液1": Value Change {
            n156 = event-data() -> ("NewVal"=w307:dbl)  [unwired: 1 in, 5 out]
            n157 = global read "多参数全局变量.vi" "MB session in"() -> (w308:refnum<class "MB_Master.lvclass">)
            n158 = call "0030H_COD_第一点标准值写入.vi"("数值"=w307, "MB session in"=w308) -> ("error out"=w309:errorcluster)  [unwired: 8 in, 1 out]
            n159 = Enqueue Element At Opposite End(queue=w304, element=T1."COD" ("枚举"), error in (no error)=w309) -> (error out=w305:errorcluster)  [unwired: 1 in, 2 out]
            n160 = call "Add State to Queue.vi"("State(s) In (\"\")"=w306) -> ("States Out"=w310:string)  [unwired: 14 in]
          }
          event "标液2": Value Change {
            n161 = event-data() -> ("NewVal"=w316:dbl)  [unwired: 1 in, 5 out]
            n162 = global read "多参数全局变量.vi" "MB session in"() -> (w317:refnum<class "MB_Master.lvclass">)
            n163 = call "0033H_COD_第二点标准值写入.vi"("数值"=w316, "MB session in"=w317) -> ("error out"=w318:errorcluster)  [unwired: 8 in, 1 out]
            n164 = Enqueue Element At Opposite End(queue=w313, element=T1."COD" ("枚举"), error in (no error)=w318) -> (error out=w314:errorcluster)  [unwired: 1 in, 2 out]
            n165 = call "Add State to Queue.vi"("State(s) In (\"\")"=w315) -> ("States Out"=w319:string)  [unwired: 14 in]
          }
          event "标液3": Value Change {
            n166 = event-data() -> ("NewVal"=w325:dbl)  [unwired: 1 in, 5 out]
            n167 = global read "多参数全局变量.vi" "MB session in"() -> (w326:refnum<class "MB_Master.lvclass">)
            n168 = call "0036H_COD_第三点标准值写入.vi"("数值"=w325, "MB session in"=w326) -> ("error out"=w327:errorcluster)  [unwired: 8 in, 1 out]
            n169 = Enqueue Element At Opposite End(queue=w322, element=T1."COD" ("枚举"), error in (no error)=w327) -> (error out=w323:errorcluster)  [unwired: 1 in, 2 out]
            n170 = call "Add State to Queue.vi"("State(s) In (\"\")"=w324) -> ("States Out"=w328:string)  [unwired: 14 in]
          }
          event "滤波设定": Value Change {
            n171 = event-data() -> ("NewVal"=w334:dbl)  [unwired: 1 in, 5 out]
            n172 = global read "多参数全局变量.vi" "MB session in"() -> (w335:refnum<class "MB_Master.lvclass">)
            n173 = call "0027H_COD_数位滤波设定写入.vi"("数值"=w334, "MB session in"=w335) -> ("error out"=w333:errorcluster)  [unwired: 8 in, 1 out]
            n174 = Enqueue Element At Opposite End(queue=w331, element=T1."COD" ("枚举"), error in (no error)=w333) -> (error out=w332:errorcluster)  [unwired: 1 in, 2 out]
            n175 = call "Add State to Queue.vi"("State(s) In (\"\")"=w336) -> ("States Out"=w337:string)  [unwired: 14 in]
          }
          event "刷新按钮": Value Change {
            n176 = event-data() -> ()  [unwired: 1 in, 6 out]
            n177 = call "Add State to Queue.vi"("State(s) In (\"\")"=w343) -> ("States Out"=w342:string)  [unwired: 14 in]
            n178 = Two Button Dialog(message="请再次确实是否恢复出厂设置！" ("消息")) -> (T button?=w340:bool)  [unwired: 2 in]
            n179 = case shown="真" w340 {
              frame False {
              }
              frame True {
                w344 = u16 33 items=["Factory Reset"=33] ("数值")
                n180 = global read "多参数全局变量.vi" "MB session in"() -> (w345:refnum<class "MB_Master.lvclass">)
                n181 = call "0026H_COD_命令寄存器写入.vi"("数值"=w344, "MB session in"=w345) -> ()  [unwired: 8 in, 2 out]
              }
            }
          }
          event "校准启动": Value Change {
            n182 = event-data() -> ()  [unwired: 1 in, 6 out]
            n183 = global read "多参数全局变量.vi" "校准运行状态"() -> (w347:T7)
            n184 = Bundle By Name(cluster=w347, "COD"=TRUE ("Turb")) -> (w348:T7)
            n185 = global write "多参数全局变量.vi" "校准运行状态"(w348) -> ()
            n186 = call "Add State to Queue.vi"("State(s) In (\"\")"=w352, "State(s) At Back (\"\")"="init: all\nCal: Place standard solution\n Cal: Calibration process\nidle" ("State(s) In (\"\")")) -> ("States Out"=w351:string)  [unwired: 13 in]
          }
          event "校准停止": Value Change {
            n187 = event-data() -> ()  [unwired: 1 in, 6 out]
            n188 = call "Add State to Queue.vi"("State(s) In (\"\")"="init: all\nCal: Over\nidle" ("State(s) In (\"\")")) -> ("States Out"=w354:string)  [unwired: 14 in]
          }
        }
      }
    }
  }
  n189 = while {
    stop <- FALSE stop-if-true
    n190 = global read "多参数全局变量.vi" "权限"() -> (w359:enum16{"一级权限", "二级权限", "三级权限"})
    n191 = Wait (ms)(milliseconds to wait=u32 1000 ("等待时间（毫秒）")) -> ()  [unwired: 1 out]
    n192 = Not Equal?(x=w359, y=enum16{"一级权限", "二级权限", "三级权限"}."一级权限") -> (x != y?=w356:bool)
    n193 = property on="滤波设定" class="DigNum (严格)"("Visible"=w356) -> ()  [unwired: 2 in, 2 out]
    n194 = property on="COD水样校正值" class="DigNum (严格)"("Visible"=w356) -> ()  [unwired: 2 in, 2 out]
    n195 = property on="COD偏移修正值" class="DigNum (严格)"("Visible"=w356) -> ()  [unwired: 2 in, 2 out]
  }
